vi "Write Instant Digital.vi"(9 "Write value group CH 8-15":u64(slide) max=255 scale=0.0..10.0, 10 "Write value group CH 0-7":u64(slide) max=255 scale=0.0..10.0, 11 "ADALM2000 Handler":u64 caption="Instrument Handle Out") -> (3 "ADALM2000 Handler 2":u64 caption="Instrument Handle Out")   [LabVIEW 2022 SP3]
uses:
  libm2k_lv.dll
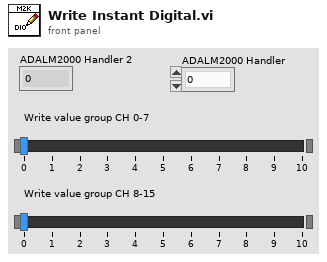
[diagram p1: front panel]
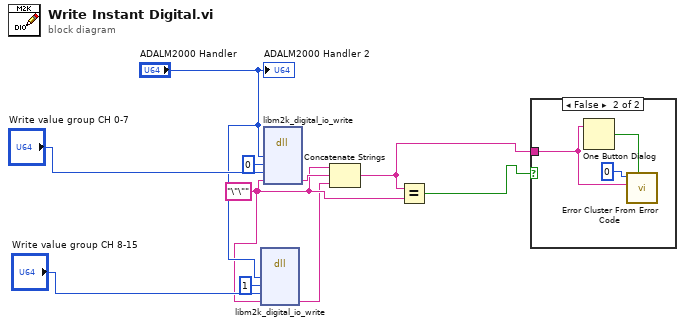
[diagram p0: block diagram]
diagram:
  w2 = "\"\""
  n1 = dll-call lib="libm2k_lv.*" fn="libm2k_digital_io_write"("instance"="ADALM2000 Handler", "groupIdx"=u64 1, "value"="Write value group CH 8-15", "err"=w2) -> ("err"=w1:string)  [unwired: 7 in, 2 out]
  n2 = dll-call lib="libm2k_lv.*" fn="libm2k_digital_io_write"("instance"="ADALM2000 Handler", "groupIdx"=u64 0, "value"="Write value group CH 0-7", "err"=w2) -> ("err"=w10:string)  [unwired: 7 in, 2 out]
  n3 = Concatenate Strings(w2, w10, w1) -> (w8:string)
  n4 = Equal?(x=w8, y=w2) -> (x = y?=w9:bool)
  n5 = case shown="False" w9 {
    tunnel: w8 -> [_ w11]
    frame True {
    }
    frame False {
      n6 = One Button Dialog(message=w11) -> (true=w13:bool)  [unwired: 1 in]
      n7 = call <vilib>:"Error Cluster From Error Code.vi"("show call chain? (False)"=w13, "error message (\"\")"=w11, "error code (0)"=0) -> ()  [unwired: 6 in, 1 out]
    }
  }
  "ADALM2000 Handler 2" <- "ADALM2000 Handler"
